vi "Configure Active Trace.vi"(5 "Format":T1, 7 "S parameter":T2(ring), 8 "error in (no error)":errorcluster, 10 "Active Trace":u8=1, 11 "VNA-CMT S2 S4 in":refnum<class "VNA-CMT S2 S4.lvclass">) -> (0 "error out":errorcluster, 3 "VNA-CMT S2 S4 out":refnum<class "VNA-CMT S2 S4.lvclass">)   [LabVIEW 2020, in "VNA-CMT S2 S4.lvclass"]
doc: "Configures the active trace.\nIt creates the trace and sets the S paramert and mode."
uses:
  VNA-CMT S2 S4.lvclass
  C:/Sandbox/Git_Sandbox/WiSpry Test Framework source code (LV20)/WiSpry Test Framework/Instruments/Instrument.lvclass
  Controls/S parm format enum.ctl
  Instrument.lvclass/Instrument.ctl
  <instrlib>/CMT S2 and S4 VNA/CMT S2 and S4 VNA.lvlib
  Instrument.lvclass
  Vector Network Analyzer.lvclass
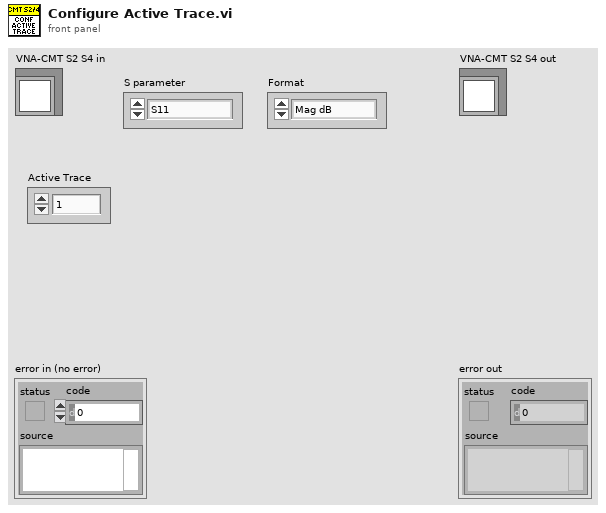
[diagram p1: front panel]
types:
  T1 = typedef "Vector Network Analyzer.lvclass/S parm format enum.ctl" = enum16{"Mag dB", "Mag", "Phase", "Smith", "Real", "Imag", "Group Delay", "SWR"}
  T2 = enum16{"S11", "S21", "S31", "S41", "S22", "S12", "S32", "S42", "S33", "S13", "S23", "S43", "S44", "S14", "S24", "S34"}
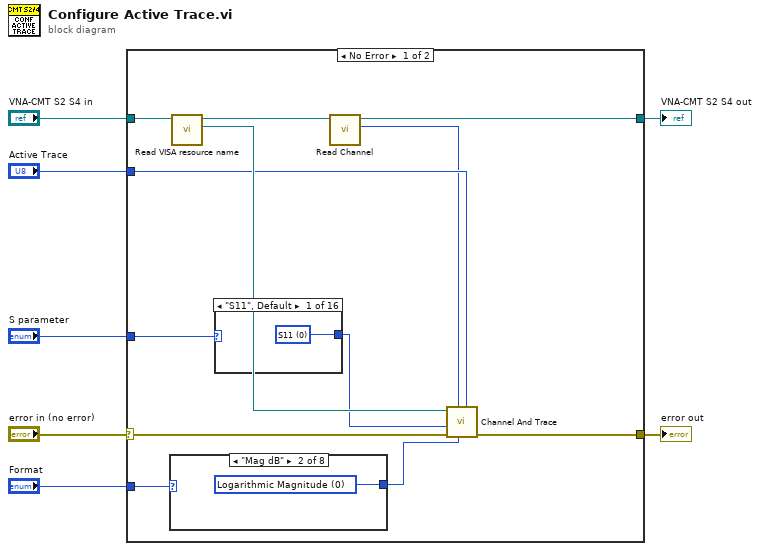
[diagram p0: block diagram]
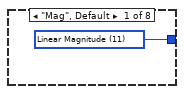
[diagram p2: hidden frame]
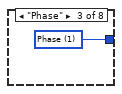
[diagram p3: hidden frame]
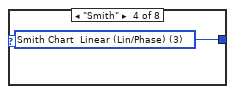
[diagram p4: hidden frame]
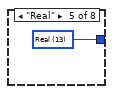
[diagram p5: hidden frame]
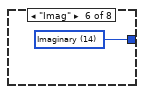
[diagram p6: hidden frame]
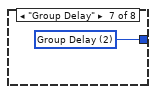
[diagram p7: hidden frame]
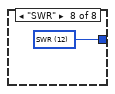
[diagram p8: hidden frame]
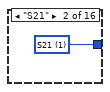
[diagram p9: hidden frame]
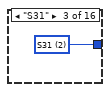
[diagram p10: hidden frame]
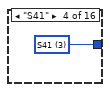
[diagram p11: hidden frame]
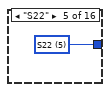
[diagram p12: hidden frame]
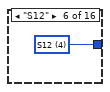
[diagram p13: hidden frame]
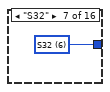
[diagram p14: hidden frame]
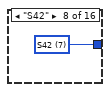
[diagram p15: hidden frame]
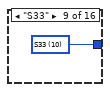
[diagram p16: hidden frame]
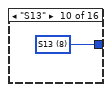
[diagram p17: hidden frame]
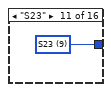
[diagram p18: hidden frame]
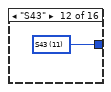
[diagram p19: hidden frame]
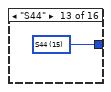
[diagram p20: hidden frame]
diagram:
  n1 = case shown="No Error" "error in (no error)" {
    selector: "error in (no error)" -> [w19 w45]
    tunnel: "VNA-CMT S2 S4 in" -> [w18 w44]
    tunnel: [w9 w44] -> w5
    tunnel: "Active Trace" -> [w16 _]
    tunnel: "S parameter" -> [w15 _]
    tunnel: "Format" -> [w13 _]
    tunnel: [w11 w45] -> w1
    frame No Error {
      n2 = case shown="\"Mag dB\"" w13 {
        tunnel: [w20 w21 w22 w23 w24 w25 w26 w27] -> w12
        frame "Mag", Default {
          w20 = u16 11 items=["Logarithmic Magnitude", "Phase", "Group Delay", "Smith Chart  Linear (Lin/Phase)", "Smith Chart  Logarithmic (Log/Phase)", "Smith Chart  Complex (Real/Imag)", "Smith Chart  Impedance (R+jX)", "Smith Chart  Admittance (G+jB)", "Polar Format (Linear)", "Polar Format (Logarithmic)", "Polar Format (Re/Im)", "Linear Magnitude", "SWR", "Real", "Imaginary", "Epanded Phase"] ("Data Format (0: Logarithmic Magnitude)")
        }
        frame "Mag dB" {
          w21 = u16 0 items=["Logarithmic Magnitude", "Phase", "Group Delay", "Smith Chart  Linear (Lin/Phase)", "Smith Chart  Logarithmic (Log/Phase)", "Smith Chart  Complex (Real/Imag)", "Smith Chart  Impedance (R+jX)", "Smith Chart  Admittance (G+jB)", "Polar Format (Linear)", "Polar Format (Logarithmic)", "Polar Format (Re/Im)", "Linear Magnitude", "SWR", "Real", "Imaginary", "Epanded Phase"] ("Data Format (0: Logarithmic Magnitude)")
        }
        frame "Phase" {
          w22 = u16 1 items=["Logarithmic Magnitude", "Phase", "Group Delay", "Smith Chart  Linear (Lin/Phase)", "Smith Chart  Logarithmic (Log/Phase)", "Smith Chart  Complex (Real/Imag)", "Smith Chart  Impedance (R+jX)", "Smith Chart  Admittance (G+jB)", "Polar Format (Linear)", "Polar Format (Logarithmic)", "Polar Format (Re/Im)", "Linear Magnitude", "SWR", "Real", "Imaginary", "Epanded Phase"] ("Data Format (0: Logarithmic Magnitude)")
        }
        frame "Smith" {
          w23 = u16 3 items=["Logarithmic Magnitude", "Phase", "Group Delay", "Smith Chart  Linear (Lin/Phase)", "Smith Chart  Logarithmic (Log/Phase)", "Smith Chart  Complex (Real/Imag)", "Smith Chart  Impedance (R+jX)", "Smith Chart  Admittance (G+jB)", "Polar Format (Linear)", "Polar Format (Logarithmic)", "Polar Format (Re/Im)", "Linear Magnitude", "SWR", "Real", "Imaginary", "Epanded Phase"] ("Data Format (0: Logarithmic Magnitude)")
        }
        frame "Real" {
          w24 = u16 13 items=["Logarithmic Magnitude", "Phase", "Group Delay", "Smith Chart  Linear (Lin/Phase)", "Smith Chart  Logarithmic (Log/Phase)", "Smith Chart  Complex (Real/Imag)", "Smith Chart  Impedance (R+jX)", "Smith Chart  Admittance (G+jB)", "Polar Format (Linear)", "Polar Format (Logarithmic)", "Polar Format (Re/Im)", "Linear Magnitude", "SWR", "Real", "Imaginary", "Epanded Phase"] ("Data Format (0: Logarithmic Magnitude)")
        }
        frame "Imag" {
          w25 = u16 14 items=["Logarithmic Magnitude", "Phase", "Group Delay", "Smith Chart  Linear (Lin/Phase)", "Smith Chart  Logarithmic (Log/Phase)", "Smith Chart  Complex (Real/Imag)", "Smith Chart  Impedance (R+jX)", "Smith Chart  Admittance (G+jB)", "Polar Format (Linear)", "Polar Format (Logarithmic)", "Polar Format (Re/Im)", "Linear Magnitude", "SWR", "Real", "Imaginary", "Epanded Phase"] ("Data Format (0: Logarithmic Magnitude)")
        }
        frame "Group Delay" {
          w26 = u16 2 items=["Logarithmic Magnitude", "Phase", "Group Delay", "Smith Chart  Linear (Lin/Phase)", "Smith Chart  Logarithmic (Log/Phase)", "Smith Chart  Complex (Real/Imag)", "Smith Chart  Impedance (R+jX)", "Smith Chart  Admittance (G+jB)", "Polar Format (Linear)", "Polar Format (Logarithmic)", "Polar Format (Re/Im)", "Linear Magnitude", "SWR", "Real", "Imaginary", "Epanded Phase"] ("Data Format (0: Logarithmic Magnitude)")
        }
        frame "SWR" {
          w27 = u16 12 items=["Logarithmic Magnitude", "Phase", "Group Delay", "Smith Chart  Linear (Lin/Phase)", "Smith Chart  Logarithmic (Log/Phase)", "Smith Chart  Complex (Real/Imag)", "Smith Chart  Impedance (R+jX)", "Smith Chart  Admittance (G+jB)", "Polar Format (Linear)", "Polar Format (Logarithmic)", "Polar Format (Re/Im)", "Linear Magnitude", "SWR", "Real", "Imaginary", "Epanded Phase"] ("Data Format (0: Logarithmic Magnitude)")
        }
      }
      n3 = call "Read VISA resource name.vi"("Instrument in"=w18) -> ("VISA resource name"=w17:refnum<visa-resource-name>, "Instrument out"=w10:refnum<class "VNA-CMT S2 S4.lvclass">)  [unwired: 9 in]
      n4 = case shown="\"S11\", Default" w15 {
        tunnel: [w28 w29 w30 w31 w32 w33 w34 w35 w36 w37 w38 w39 w40 w41 w42 w43] -> w14
        frame "S11", Default {
          w28 = u16 0 items=["S11", "S21", "S31", "S41", "S12", "S22", "S32", "S42", "S13", "S23", "S33", "S43", "S14", "S24", "S34", "S44", "A", "B", "C", "D", "R1", "R2", "R3", "R4", "T1", "T2", "T3", "T4"] ("Measurement Parameters (0: S11)")
        }
        frame "S21" {
          w29 = u16 1 items=["S11", "S21", "S31", "S41", "S12", "S22", "S32", "S42", "S13", "S23", "S33", "S43", "S14", "S24", "S34", "S44", "A", "B", "C", "D", "R1", "R2", "R3", "R4", "T1", "T2", "T3", "T4"] ("Measurement Parameters (0: S11)")
        }
        frame "S31" {
          w30 = u16 2 items=["S11", "S21", "S31", "S41", "S12", "S22", "S32", "S42", "S13", "S23", "S33", "S43", "S14", "S24", "S34", "S44", "A", "B", "C", "D", "R1", "R2", "R3", "R4", "T1", "T2", "T3", "T4"] ("Measurement Parameters (0: S11)")
        }
        frame "S41" {
          w31 = u16 3 items=["S11", "S21", "S31", "S41", "S12", "S22", "S32", "S42", "S13", "S23", "S33", "S43", "S14", "S24", "S34", "S44", "A", "B", "C", "D", "R1", "R2", "R3", "R4", "T1", "T2", "T3", "T4"] ("Measurement Parameters (0: S11)")
        }
        frame "S22" {
          w32 = u16 5 items=["S11", "S21", "S31", "S41", "S12", "S22", "S32", "S42", "S13", "S23", "S33", "S43", "S14", "S24", "S34", "S44", "A", "B", "C", "D", "R1", "R2", "R3", "R4", "T1", "T2", "T3", "T4"] ("Measurement Parameters (0: S11)")
        }
        frame "S12" {
          w33 = u16 4 items=["S11", "S21", "S31", "S41", "S12", "S22", "S32", "S42", "S13", "S23", "S33", "S43", "S14", "S24", "S34", "S44", "A", "B", "C", "D", "R1", "R2", "R3", "R4", "T1", "T2", "T3", "T4"] ("Measurement Parameters (0: S11)")
        }
        frame "S32" {
          w34 = u16 6 items=["S11", "S21", "S31", "S41", "S12", "S22", "S32", "S42", "S13", "S23", "S33", "S43", "S14", "S24", "S34", "S44", "A", "B", "C", "D", "R1", "R2", "R3", "R4", "T1", "T2", "T3", "T4"] ("Measurement Parameters (0: S11)")
        }
        frame "S42" {
          w35 = u16 7 items=["S11", "S21", "S31", "S41", "S12", "S22", "S32", "S42", "S13", "S23", "S33", "S43", "S14", "S24", "S34", "S44", "A", "B", "C", "D", "R1", "R2", "R3", "R4", "T1", "T2", "T3", "T4"] ("Measurement Parameters (0: S11)")
        }
        frame "S33" {
          w36 = u16 10 items=["S11", "S21", "S31", "S41", "S12", "S22", "S32", "S42", "S13", "S23", "S33", "S43", "S14", "S24", "S34", "S44", "A", "B", "C", "D", "R1", "R2", "R3", "R4", "T1", "T2", "T3", "T4"] ("Measurement Parameters (0: S11)")
        }
        frame "S13" {
          w37 = u16 8 items=["S11", "S21", "S31", "S41", "S12", "S22", "S32", "S42", "S13", "S23", "S33", "S43", "S14", "S24", "S34", "S44", "A", "B", "C", "D", "R1", "R2", "R3", "R4", "T1", "T2", "T3", "T4"] ("Measurement Parameters (0: S11)")
        }
        frame "S23" {
          w38 = u16 9 items=["S11", "S21", "S31", "S41", "S12", "S22", "S32", "S42", "S13", "S23", "S33", "S43", "S14", "S24", "S34", "S44", "A", "B", "C", "D", "R1", "R2", "R3", "R4", "T1", "T2", "T3", "T4"] ("Measurement Parameters (0: S11)")
        }
        frame "S43" {
          w39 = u16 11 items=["S11", "S21", "S31", "S41", "S12", "S22", "S32", "S42", "S13", "S23", "S33", "S43", "S14", "S24", "S34", "S44", "A", "B", "C", "D", "R1", "R2", "R3", "R4", "T1", "T2", "T3", "T4"] ("Measurement Parameters (0: S11)")
        }
        frame "S44" {
          w40 = u16 15 items=["S11", "S21", "S31", "S41", "S12", "S22", "S32", "S42", "S13", "S23", "S33", "S43", "S14", "S24", "S34", "S44", "A", "B", "C", "D", "R1", "R2", "R3", "R4", "T1", "T2", "T3", "T4"] ("Measurement Parameters (0: S11)")
        }
        frame "S14" {
          w41 = u16 12 items=["S11", "S21", "S31", "S41", "S12", "S22", "S32", "S42", "S13", "S23", "S33", "S43", "S14", "S24", "S34", "S44", "A", "B", "C", "D", "R1", "R2", "R3", "R4", "T1", "T2", "T3", "T4"] ("Measurement Parameters (0: S11)")
        }
        frame "S24" {
          w42 = u16 13 items=["S11", "S21", "S31", "S41", "S12", "S22", "S32", "S42", "S13", "S23", "S33", "S43", "S14", "S24", "S34", "S44", "A", "B", "C", "D", "R1", "R2", "R3", "R4", "T1", "T2", "T3", "T4"] ("Measurement Parameters (0: S11)")
        }
        frame "S34" {
          w43 = u16 14 items=["S11", "S21", "S31", "S41", "S12", "S22", "S32", "S42", "S13", "S23", "S33", "S43", "S14", "S24", "S34", "S44", "A", "B", "C", "D", "R1", "R2", "R3", "R4", "T1", "T2", "T3", "T4"] ("Measurement Parameters (0: S11)")
        }
      }
      n5 = call-dynamic "Read Channel.vi"("Vector Network Analyzer in"=w10) -> ("Channel"=w8:i32, "Vector Network Analyzer out"=w9:refnum<class "VNA-CMT S2 S4.lvclass">)  [unwired: 9 in]
      n6 = call <instrlib>:"Channel And Trace.vi"("Active Trace (1)"=w16, "Data Format (0: Logarithmic Magnitude)"=w12, "Active Channel (1)"=w8, "error in (no error)"=w19, "Measurement Parameters (0: S11)"=w14, "VISA resource name"=w17) -> ("error out"=w11:errorcluster)  [unwired: 4 in, 1 out]
    }
    frame Error {
    }
  }
  "error out" <- w1
  "VNA-CMT S2 S4 out" <- w5
